vi "Serialize.vi"(7 "MsgSerializer":refnum<class "MsgSerializer.lvclass">, 8 "error in (no error)":errorcluster, 11 "Value":variant) -> (0 "error out":errorcluster, 3 "Serialized Message":string)   [LabVIEW 2013, in "Caraya.lvlib" / "MsgSerializer.lvclass"]
uses:
  MsgSerializer.lvclass
  MsgSerializer.lvclass/MsgSerializer.ctl
  <vilib>/Utility/VariantDataType/VariantType.lvlib
  Caraya.lvlib
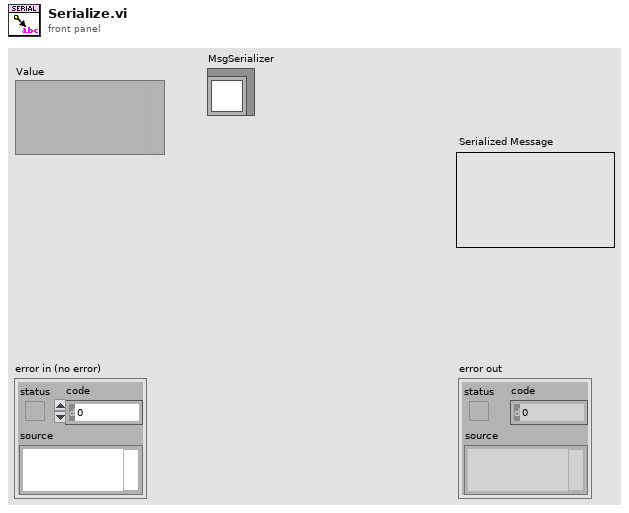
[diagram p1: front panel]
types:
  T1 = typedef "VariantType.lvlib/Type.ctl" = enum8{"Invalid Type", "Void", "I8", "I16", "I32", "I64", "U8", "U16", "U32", "U64", "Single Float", "Double Float", "Extended Float", "Single Complex", "Double Complex", "Extended Complex", "Enum U8", "Enum U16", "Enum U32", "Enum U64", "Single Float With Unit", "Double Float With Unit", "Extended Float With Unit", "Single Complex with Unit", "Double Complex with Unit", "Extended Complex with Unit", "Boolean", "String", "Path", "Picture", "Tag", "Array", "Cluster", "Variant", "LV Variant", "Waveform", "Timestamp", "Digital Waveform", "Digital Data", "ExpressData", "Refnum", "External Data", "VI", "Poly VI", "LabVIEW Class Instance", "Fixed Point"}
  T2 = typedef "Caraya.lvlib/MsgSerializer.lvclass/decimal-notation -- enum.ctl" = enum16{"System-defined", "dot-notation", "comma-notation"}
  T3 = typedef "TD_MDTFlavor.ctl" = enum16{"kUnknown", "OldDblWaveform", "I16Waveform", "DBLWaveform", "Unused(4)", "SGLWaveform", "Timestamp", "DigitalTable", "DigitalWaveform", "Dynamic Express", "ExtWaveform", "U8Waveform", "U16Waveform", "U32Waveform", "I8Waveform", "I32Waveform", "CSGWaveform", "CDBWaveform", "CXTWaveform", "I64Waveform", "U64Waveform"}
  T4 = typedef "VariantType.lvlib/RefnumType.ctl" = enum16{"NotARefnum", "UnknownRefnum", "Generic", "Datalog", "ByteStream", "Device", "Occurence", "TCPNetConnection", "Auto", "Menu", "Imaq", "Hardware", "DataSocket", "Visa", "IVI", "UDPNetConnection", "Notifier", "Queue", "Irda", "EventReg", "DotNet", "UserEvent", "Callback", "UNUSED_EMPTY_POSITION", "BlueToothNetConnection", "LVObjApp", "LVObjVI", "LVObjUnknown", "GenericClass", "UserDefinedRefnumTag", "DataValue", "RT FIFO", "TDMS File"}
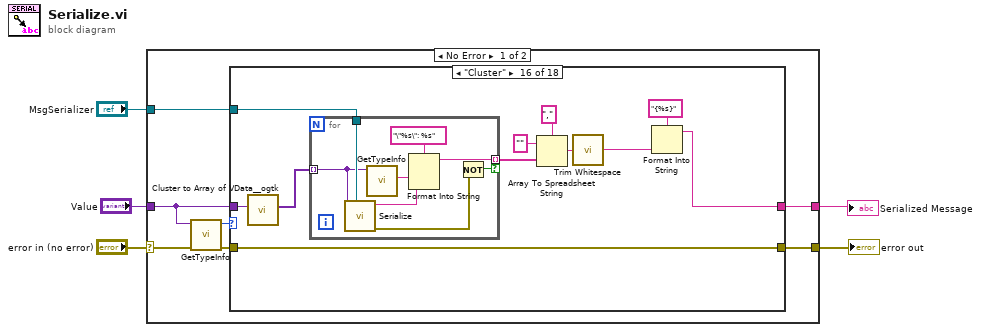
[diagram p0: block diagram]
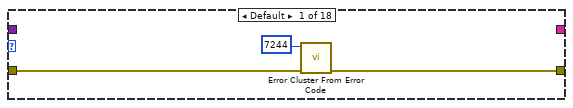
[diagram p2: hidden frame]
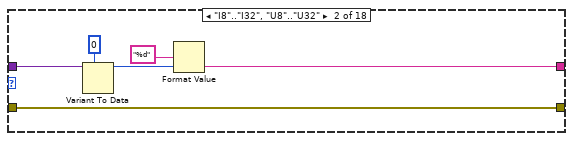
[diagram p3: hidden frame]
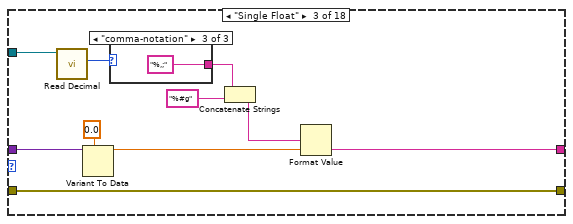
[diagram p4: hidden frame]
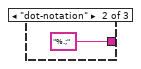
[diagram p6: hidden frame]
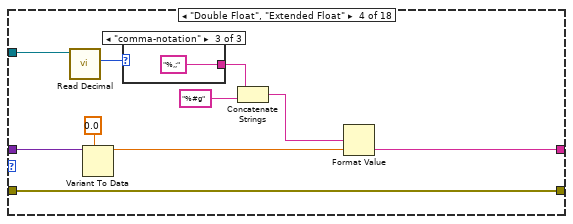
[diagram p7: hidden frame]
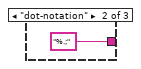
[diagram p9: hidden frame]
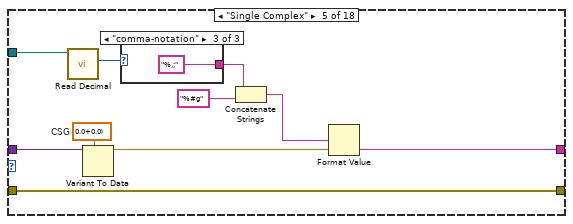
[diagram p10: hidden frame]
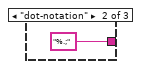
[diagram p12: hidden frame]
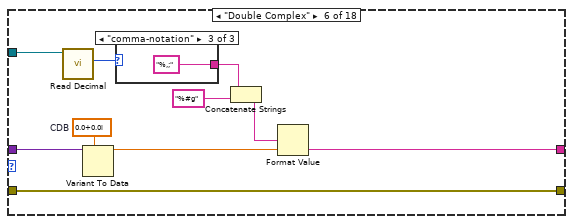
[diagram p13: hidden frame]
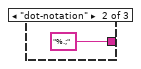
[diagram p15: hidden frame]
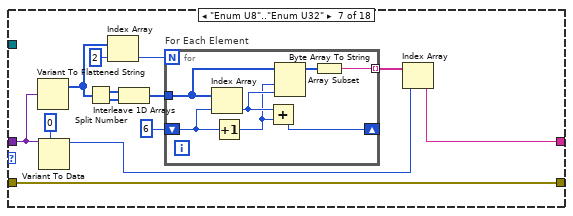
[diagram p16: hidden frame]
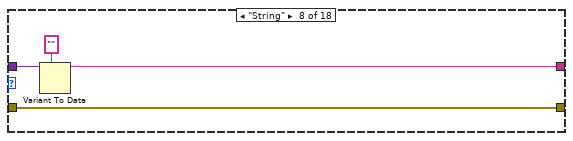
[diagram p17: hidden frame]
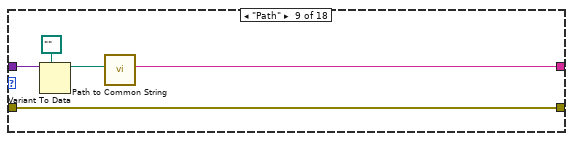
[diagram p18: hidden frame]
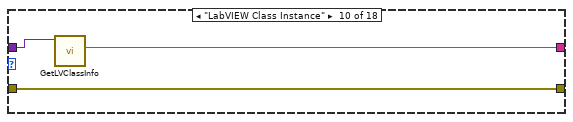
[diagram p19: hidden frame]
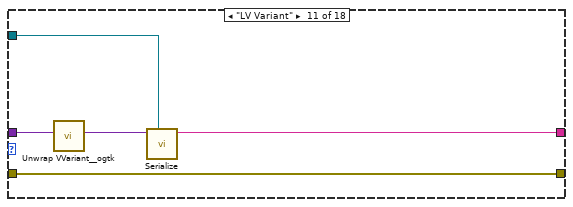
[diagram p20: hidden frame]
diagram:
  n1 = case shown="No Error" "error in (no error)" {
    selector: "error in (no error)" -> [w7 w213]
    tunnel: "MsgSerializer" -> [w12 _]
    tunnel: [w11 _] -> w4
    tunnel: "Value" -> [w10 _]
    tunnel: [w8 w213] -> w2
    frame No Error {
      n2 = call <vilib>:"GetTypeInfo.vi"("error in (no error)"=w7, "Variant"=w10) -> ("error out"=w6:errorcluster, "Type Enum"=w9:T1)  [unwired: 5 in, 3 out]
      n3 = case shown="\"Cluster\"" w9 {
        tunnel: [_ w17 w28 w40 w53 w65 w70 w90 w94 w99 w103 w107 w121 w128 w146 w158 w180 w203] -> w11
        tunnel: w10 -> [_ w21 w31 w43 w55 w67 w73 w92 w97 w101 w104 w110 w125 w129 w150 w155 w178 w199]
        tunnel: w12 -> [_ _ w26 w35 w47 w59 _ _ _ _ w102 _ _ _ _ w162 w179 w207]
        tunnel: w6 -> [w14 w16 w27 w39 w51 w63 w71 w91 w95 w100 w106 w109 w124 w127 w145 w154 w171 w197]
        tunnel: [w13 w16 w27 w39 w51 w63 w71 w91 w95 w100 w106 w108 w124 w126 w145 w154 w171 w197] -> w8
        frame Default {
          n4 = call <vilib>:"Error Cluster From Error Code.vi"("error in (no error)"=w14, "error code (0)"=7244) -> ("error out"=w13:errorcluster)  [unwired: 7 in]
        }
        frame "I8".."I32", "U8".."U32" {
          n5 = Variant To Data(type=i64 0, Variant=w21) -> (data=w20:i64)  [unwired: 1 in, 1 out]
          n6 = Format Value(format string="%d", value (0)=w20) -> (output string=w17:string)  [unwired: 1 in]
        }
        frame "Single Float" {
          n7 = call "Read Decimal.vi"("MsgSerializer"=w26) -> ("Decimal"=w25:T2)  [unwired: 9 in, 1 out]
          n8 = Variant To Data(type=sgl 0.0, Variant=w31) -> (data=w30:sgl)  [unwired: 1 in, 1 out]
          n9 = case shown="\"comma-notation\"" w25 {
            tunnel: [_ "%.;" ("format string") "%,;" ("format string")] -> w24
            frame "System-defined", Default {
            }
            frame "dot-notation" {
            }
            frame "comma-notation" {
            }
          }
          n10 = Concatenate Strings(w24, "%#g" ("format string")) -> (w22:string)
          n11 = Format Value(format string=w22, value (0)=w30) -> (output string=w28:string)  [unwired: 1 in]
        }
        frame "Double Float", "Extended Float" {
          n12 = call "Read Decimal.vi"("MsgSerializer"=w35) -> ("Decimal"=w38:T2)  [unwired: 9 in, 1 out]
          n13 = Variant To Data(type=0.0, Variant=w43) -> (data=w42:dbl)  [unwired: 1 in, 1 out]
          n14 = case shown="\"comma-notation\"" w38 {
            tunnel: [_ "%.;" ("format string") "%,;" ("format string")] -> w37
            frame "System-defined", Default {
            }
            frame "dot-notation" {
            }
            frame "comma-notation" {
            }
          }
          n15 = Concatenate Strings(w37, "%#g" ("format string")) -> (w34:string)
          n16 = Format Value(format string=w34, value (0)=w42) -> (output string=w40:string)  [unwired: 1 in]
        }
        frame "Single Complex" {
          w52 = csg 0.0+0.0i  # CSG
          n17 = call "Read Decimal.vi"("MsgSerializer"=w47) -> ("Decimal"=w50:T2)  [unwired: 9 in, 1 out]
          n18 = Variant To Data(type=w52, Variant=w55) -> (data=w54:csg)  [unwired: 1 in, 1 out]
          n19 = case shown="\"comma-notation\"" w50 {
            tunnel: [_ "%.;" ("format string") "%,;" ("format string")] -> w49
            frame "System-defined", Default {
            }
            frame "dot-notation" {
            }
            frame "comma-notation" {
            }
          }
          n20 = Concatenate Strings(w49, "%#g" ("format string")) -> (w46:string)
          n21 = Format Value(format string=w46, value (0)=w54) -> (output string=w53:string)  [unwired: 1 in]
        }
        frame "Double Complex" {
          w64 = cdb 0.0+0.0i  # CDB
          n22 = call "Read Decimal.vi"("MsgSerializer"=w59) -> ("Decimal"=w62:T2)  [unwired: 9 in, 1 out]
          n23 = Variant To Data(type=w64, Variant=w67) -> (data=w66:cdb)  [unwired: 1 in, 1 out]
          n24 = case shown="\"comma-notation\"" w62 {
            tunnel: [_ "%.;" ("format string") "%,;" ("format string")] -> w61
            frame "System-defined", Default {
            }
            frame "dot-notation" {
            }
            frame "comma-notation" {
            }
          }
          n25 = Concatenate Strings(w61, "%#g" ("format string")) -> (w58:string)
          n26 = Format Value(format string=w58, value (0)=w66) -> (output string=w65:string)  [unwired: 1 in]
        }
        frame "Enum U8".."Enum U32" {
          n27 = Variant To Flattened String(Variant=w73) -> (1:w74:i16[])  [unwired: 1 out]
          n28 = Variant To Data(type=u32 0, Variant=w73) -> (data=w72:u32)  [unwired: 1 in, 1 out]
          n29 = Split Number(x=w74) -> (hi(x)=w79:u8[], lo(x)=w78:u8[])
          n30 = Index Array(array=w74, index=2) -> (element=w81:i16)
          n31 = Interleave 1D Arrays(w79, w78) -> (w77:u8[])
          n32 = for "For Each Element" {
            N: w81 -> [_]
            shift-right: [w86] -> _
            shift-left: 6 ("index") -> [w89]
            tunnel: w77 -> [w87]
            tunnel: [w84] -> w75 mode=indexing
            n33 = Index Array(array=w87, index=w89) -> (element=w85:u8)
            n34 = Increment(x=w89) -> (x+1=w83:i32)
            n35 = Add(x=w85, y=w83) -> (x+y=w86:i32)
            n36 = Array Subset(array=w87, index=w83, length=w85) -> (w88:u8[])
            n37 = Byte Array To String(unsigned byte array=w88) -> (string=w84:string)
          }
          n38 = Index Array(array=w75, index=w72) -> (element=w70:string)
        }
        frame "String" {
          n39 = Variant To Data(type="", Variant=w92) -> (data=w90:string)  [unwired: 1 in, 1 out]
        }
        frame "Path" {
          n40 = Variant To Data(type=path "", Variant=w97) -> (data=w96:path)  [unwired: 1 in, 1 out]
          n41 = call "Path to Common String.vi"("specific path"=w96) -> ("common path"=w94:string)  [unwired: 10 in]
        }
        frame "LabVIEW Class Instance" {
          n42 = call <vilib>:"GetLVClassInfo.vi"("Variant"=w101) -> ("LV Class File Name"=w99:string)  [unwired: 8 in, 2 out]
        }
        frame "LV Variant" {
          n43 = call <userlib>:"Unwrap VVariant__ogtk.vi"("VVariant"=w104) -> ("Variant"=w105:variant)  [unwired: 9 in, 1 out]
          n44 = call-dynamic "Serialize.vi"("MsgSerializer"=w102, "Value"=w105) -> ("Serialized Message"=w103:string)  [unwired: 8 in, 1 out]
        }
        frame "Waveform" {
          n45 = Variant To Flattened String(Variant=w110) -> (1:w112:i16[])  [unwired: 1 out]
          n46 = call <vilib>:"TD_Get MDT Information.vi"("Type descriptor"=w112) -> ("MDT Flavor"=w111:T3)  [unwired: 9 in, 1 out]
          n47 = case shown="\"Timestamp\"" w111 {
            tunnel: w110 -> [_ w119]
            tunnel: [_ w116] -> w107
            tunnel: w109 -> [w114 w118]
            tunnel: [w115 w118] -> w108
            frame Default {
              n48 = call <vilib>:"Error Cluster From Error Code.vi"("error in (no error)"=w114, "error code (0)"=7244) -> ("error out"=w115:errorcluster)  [unwired: 7 in]
            }
            frame "Timestamp" {
              n49 = Variant To Data(type=timestamp(0 s since 1904-01-01) ("current time"), Variant=w119) -> (data=w117:timestamp)  [unwired: 1 in, 1 out]
              n50 = call <vilib>:"Timestamp to ISO8601 UTC DateTime.vi"("Timestamp (now)"=w117) -> ("ISO8601 UTC DateTime"=w116:string)  [unwired: 10 in]
            }
          }
        }
        frame "Timestamp" {
          n51 = Variant To Data(type=timestamp(0 s since 1904-01-01) ("current time"), Variant=w125) -> (data=w122:timestamp)  [unwired: 1 in, 1 out]
          n52 = call <vilib>:"Timestamp to ISO8601 UTC DateTime.vi"("Timestamp (now)"=w122) -> ("ISO8601 UTC DateTime"=w121:string)  [unwired: 10 in]
        }
        frame "Refnum" {
          n53 = call <vilib>:"GetRefnumInfo.vi"("Variant"=w129) -> ("ReferenceType"=w130:T4)  [unwired: 7 in, 3 out]
          n54 = case shown="Default" w130 {
            tunnel: w129 -> [w139 w143]
            tunnel: [w137 w140] -> w128
            tunnel: w127 -> [w136 w142]
            tunnel: [w135 w141] -> w126
            frame Default {
              n55 = Variant To Data(error in=w136, type=refnum<k0> refnum, Variant=w139) -> (data=w131:refnum<k0>, error out=w135:errorcluster)
              n56 = Type Cast(type=u32 0, x=w131) -> (*(type *) &x=w132:u32)
              n57 = Format Value(format string="%d", value (0)=w132) -> (output string=w137:string)  [unwired: 1 in]
            }
            frame "Visa", "IVI" {
              n58 = Variant To Data(error in=w142, type="", Variant=w143) -> (data=w140:string, error out=w141:errorcluster)
            }
          }
        }
        frame "Boolean" {
          n59 = Variant To Data(type=FALSE, Variant=w150) -> (data=w147:bool)  [unwired: 1 in, 1 out]
          n60 = Select(t="true", s=w147, f="false") -> (s? t:f=w146:string)
        }
        frame "Cluster" {
          n61 = call <userlib>:"Cluster to Array of VData__ogtk.vi"("Cluster"=w155) -> ("Array of VData"=w152:variant[])  [unwired: 9 in, 1 out]
          n62 = for {
            tunnel: w152 -> [w166] mode=indexing
            tunnel: w162 -> [w169]
            tunnel: [w167] -> w153 mode=indexing if=w163
            n63 = call-dynamic "Serialize.vi"("MsgSerializer"=w169, "Value"=w166) -> ("error out"=w164:errorcluster, "Serialized Message"=w170:string)  [unwired: 8 in]
            n64 = call <vilib>:"GetTypeInfo.vi"("Variant"=w166) -> ("Name"=w165:string)  [unwired: 6 in, 4 out]
            n65 = Format Into String(format string="\"%s\": %s", w165, w170) -> (resulting string=w167:string)  [unwired: 2 in, 1 out]
            n66 = Not(x=w164) -> (.not. x?=w163:bool)
          }
          n67 = Array To Spreadsheet String(delimiter (Tab)=",", array=w153, 3:"" ("format string")) -> (spreadsheet string=w161:string)
          n68 = call <vilib>:"Trim Whitespace.vi"("string"=w161) -> ("trimmed string"=w160:string)  [unwired: 1 in]
          n69 = Format Into String(format string="{%s}", w160) -> (resulting string=w158:string)  [unwired: 2 in, 1 out]
        }
        frame "Void" {
          n70 = Get Variant Attribute(Variant=w178) -> (names=w176:string[], values=w175:variant[])  [unwired: 3 in, 2 out]
          n71 = Empty Array?(array=w176) -> (empty?=w177:bool)
          n72 = case shown="False" w177 {
            tunnel: w176 -> [w186 _]
            tunnel: w175 -> [w187 _]
            tunnel: w179 -> [w188 _]
            tunnel: [w181 _] -> w172
            frame False {
              n73 = for {
                tunnel: w188 -> [w196]
                tunnel: w187 -> [w195] mode=indexing
                tunnel: w186 -> [w194] mode=indexing
                tunnel: [w191] -> w182 mode=indexing if=w189
                n74 = call-dynamic "Serialize.vi"("MsgSerializer"=w196, "Value"=w195) -> ("error out"=w190:errorcluster, "Serialized Message"=w193:string)  [unwired: 8 in]
                n75 = Not(x=w190) -> (.not. x?=w189:bool)
                n76 = Format Into String(format string="\"%s\": %s", w194, w193) -> (resulting string=w191:string)  [unwired: 2 in, 1 out]
              }
              n77 = Array To Spreadsheet String(delimiter (Tab)=",", array=w182, 3:"" ("format string")) -> (spreadsheet string=w185:string)
              n78 = call <vilib>:"Trim Whitespace.vi"("string"=w185) -> ("trimmed string"=w181:string)  [unwired: 1 in]
            }
            frame True {
            }
          }
          n79 = Concatenate Strings("{" ("string"), w172, "}" ("format string")) -> (w180:string)
        }
        frame "Array" {
          n80 = call <userlib>:"Array to Array of VData__ogtk.vi"("MultiD Array"=w199) -> ("1D Array of Variants"=w198:variant[])  [unwired: 9 in, 1 out]
          n81 = for {
            tunnel: w198 -> [w211] mode=indexing
            tunnel: w207 -> [w212]
            tunnel: [w210] -> w200 mode=indexing if=w209
            n82 = call-dynamic "Serialize.vi"("MsgSerializer"=w212, "Value"=w211) -> ("error out"=w208:errorcluster, "Serialized Message"=w210:string)  [unwired: 8 in]
            n83 = Not(x=w208) -> (.not. x?=w209:bool)
          }
          n84 = Array To Spreadsheet String(delimiter (Tab)=",", array=w200, 3:"" ("format string")) -> (spreadsheet string=w206:string)
          n85 = call <vilib>:"Trim Whitespace.vi"("string"=w206) -> ("trimmed string"=w205:string)  [unwired: 1 in]
          n86 = Format Into String(format string="[%s]", w205) -> (resulting string=w203:string)  [unwired: 2 in, 1 out]
        }
      }
    }
    frame Error {
    }
  }
  "error out" <- w2
  "Serialized Message" <- w4
